vi "Temperature Bath - Simple Controller.vi"() -> ()   [LabVIEW 2023]
uses:
  <vilib>/Utility/error.llb/Trim Whitespace One-Sided.vi
  <vilib>/Instr/_visa.llb/VISA Configure Serial Port (Instr).vi
  <vilib>/Utility/file.llb/Write Delimited Spreadsheet (string).vi
panel:
  in  "stop":bool
  in  "format (%s)":string="%s"
  in  "delimiter (\\t)":string="\t"
  out "error out":errorcluster
  in  "Boolean 3":bool
  in  "VISA resource name 2":refnum<visa-resource-name>
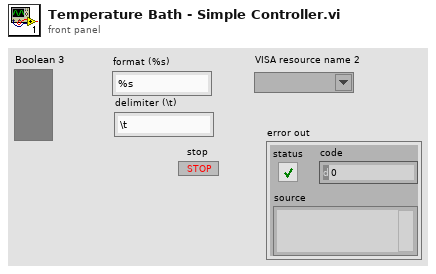
[diagram p1: front panel]
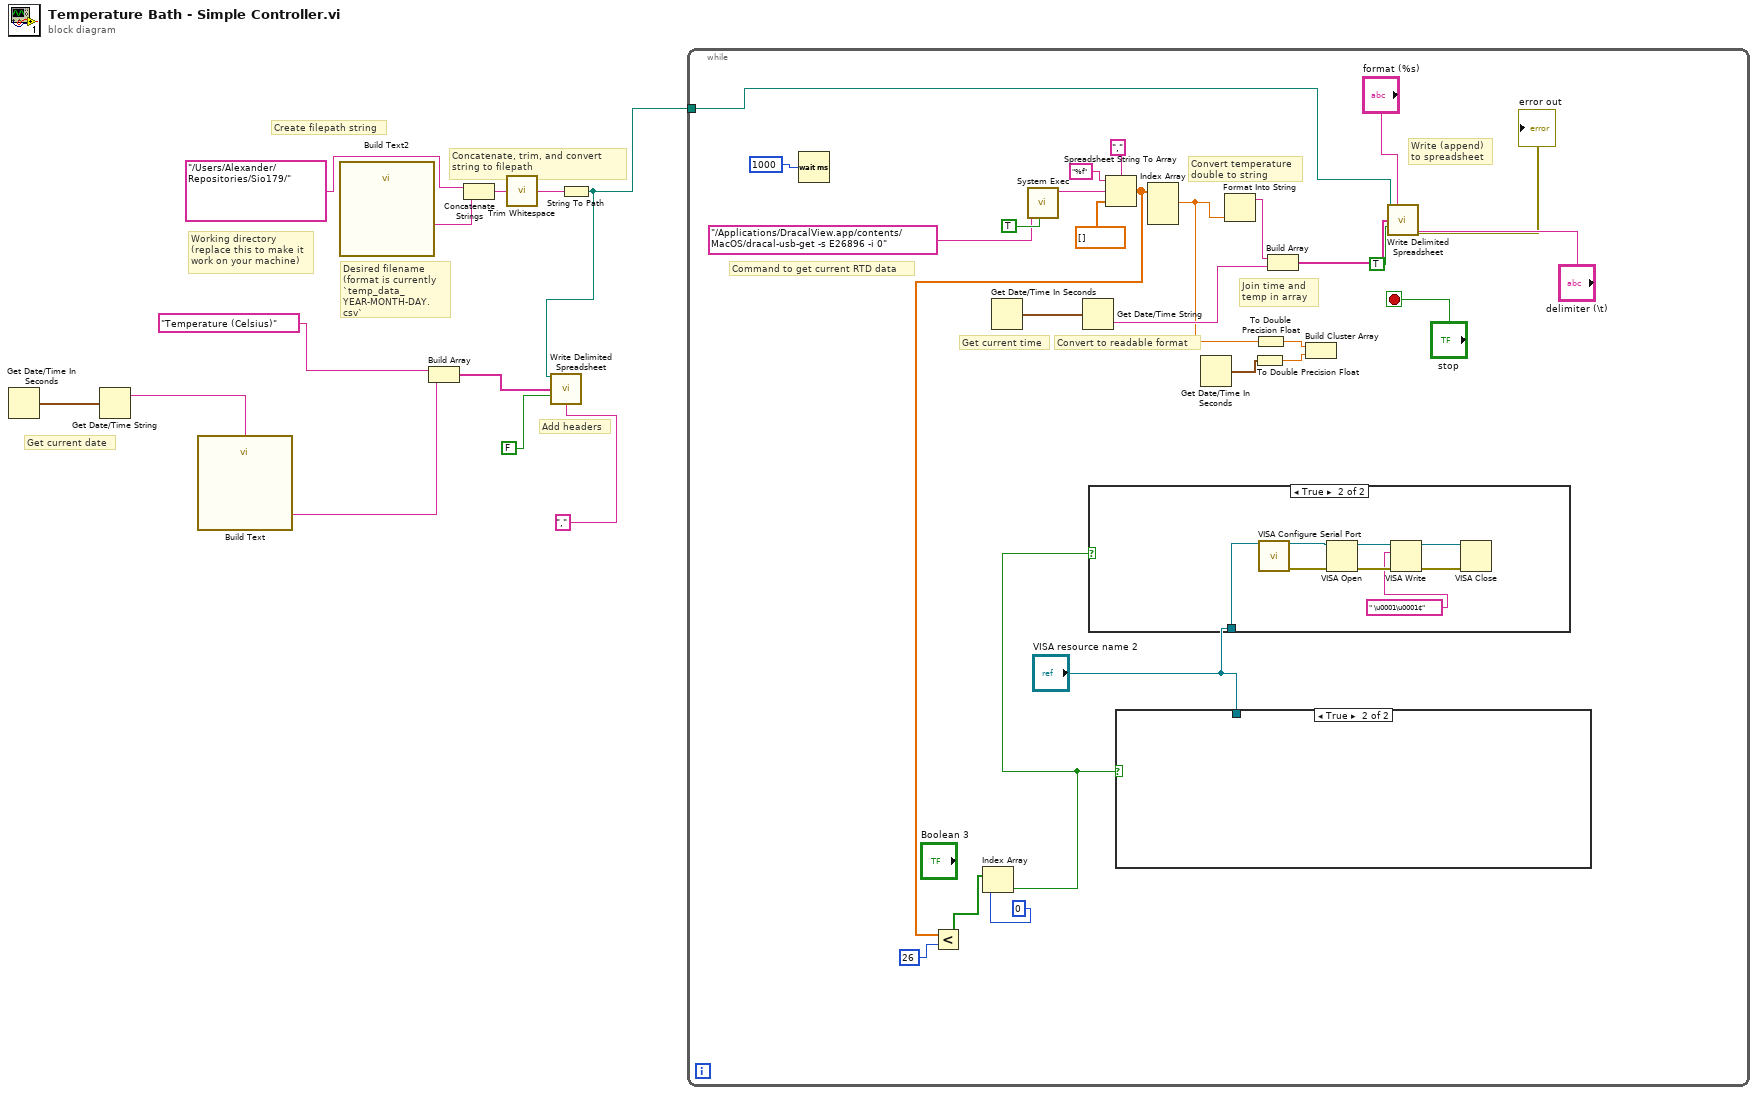
[diagram p0: block diagram]
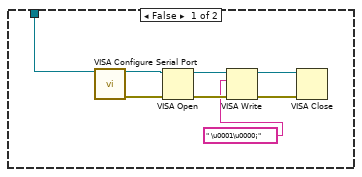
[diagram p2: hidden frame]
diagram:
  # "Add headers"
  # "Get current date"
  # "Concatenate, trim, and convert string to filepath"
  # "Desired filename (format is currently `temp_data_YEAR-MONTH-DAY.csv`"
  # "Working directory (replace this to make it work on your machine)"
  # "Create filepath string"
  n1 = Get Date/Time In Seconds() -> (seconds since 1Jan1904=w10:timestamp)
  n2 = Get Date/Time String(seconds (now)=w10) -> (date string=w6:string)  [unwired: 2 in, 1 out]
  n3 = call "Build Text"("date"=w6) -> ("Result"=w9:string)  [unwired: 13 in, 1 out]
  n4 = call "Build Text2"() -> ("Result"=w5:string)  [unwired: 14 in, 1 out]
  n5 = Build Array("Temperature (Celsius)", w9) -> (w8:string[])
  n6 = Concatenate Strings("/Users/Alexander/Repositories/Sio179/", w5) -> (w11:string)
  n7 = call <vilib>:"Trim Whitespace.vi"("string"=w11) -> ("trimmed string"=w12:string)  [unwired: 1 in]
  n8 = String To Path(string=w12) -> (path=w7:path)
  n9 = call-poly <vilib>:"Write Delimited Spreadsheet.vi"("file path (dialog if empty)"=w7, "1D data"=w8, "append to file? (new file:F)"=FALSE, "delimiter (\\t)"=",") -> ()  [unwired: 10 in, 2 out]
  n10 = while {
    tunnel: w7 -> [w23]
    stop <- "stop" stop-if-true
    # "Command to get current RTD data"
    # "Join time and temp in array"
    # "Convert temperature double to string"
    # "Convert to readable format"
    # "Get current time"
    # "Write (append) to spreadsheet"
    n11 = Wait (ms)(milliseconds to wait=u32 1000) -> ()  [unwired: 1 out]
    n12 = Get Date/Time In Seconds() -> (seconds since 1Jan1904=w32:timestamp)
    n13 = call <vilib>:"System Exec.vi"("run minimized? (F)"=TRUE, "command line"="/Applications/DracalView.app/contents/MacOS/dracal-usb-get -s E26896 -i 0") -> ("standard output"=w35:string)  [unwired: 6 in, 3 out]
    n14 = Get Date/Time String(seconds (now)=w32) -> (time string=w33:string)  [unwired: 2 in, 1 out]
    n15 = Spreadsheet String To Array(delimiter (Tab)=",", format string="%f", spreadsheet string=w35, array type (2D Dbl)=dbl[] [] ("Array")) -> (array=w18:dbl[])
    n16 = Less?(x=w18, y=26) -> (x < y?=w16:bool[])
    n17 = Index Array(array=w16, index=0) -> (element=w17:bool)
    n18 = case shown="True" w17 {
      tunnel: "VISA resource name 2" -> [_ w48]
      frame False {
      }
      frame True {
        n19 = call-poly "VISA Configure Serial Port"("VISA resource name"=w48) -> ("VISA resource name out"=w55:refnum<visa-resource-name>, "error out"=w54:errorcluster)  [unwired: 13 in]
        n20 = VISA Open(error in (no error)=w54, VISA resource name=w55) -> (VISA resource name=w53:refnum<visa-resource-name>, error out=w52:errorcluster)  [unwired: 3 in]
        n21 = VISA Write(VISA resource name=w53, write buffer=" \u0001\u0001¢", error in (no error)=w52) -> (VISA resource name out=w51:refnum<visa-resource-name>, error out=w50:errorcluster)  [unwired: 1 out]
        n22 = VISA Close(VISA resource name=w51, error in (no error)=w50) -> ()  [unwired: 1 out]
      }
    }
    n23 = case shown="True" w17 {
      tunnel: "VISA resource name 2" -> [w40 _]
      frame False {
        n24 = call-poly "VISA Configure Serial Port"("VISA resource name"=w40) -> ("VISA resource name out"=w47:refnum<visa-resource-name>, "error out"=w46:errorcluster)  [unwired: 13 in]
        n25 = VISA Open(error in (no error)=w46, VISA resource name=w47) -> (VISA resource name=w45:refnum<visa-resource-name>, error out=w44:errorcluster)  [unwired: 3 in]
        n26 = VISA Write(VISA resource name=w45, write buffer=" \u0001\u0000¡", error in (no error)=w44) -> (VISA resource name out=w43:refnum<visa-resource-name>, error out=w42:errorcluster)  [unwired: 1 out]
        n27 = VISA Close(VISA resource name=w43, error in (no error)=w42) -> ()  [unwired: 1 out]
      }
      frame True {
      }
    }
    n28 = Index Array(array=w18) -> (element #1=w22:dbl)  [unwired: 3 in, 2 out]
    n29 = Get Date/Time In Seconds() -> (seconds since 1Jan1904=w21:timestamp)
    n30 = Format Into String(w22) -> (resulting string=w24:string)  [unwired: 3 in, 1 out]
    n31 = To Double Precision Float(number=w21) -> (double precision float=w19:dbl)
    n32 = To Double Precision Float(number=w22) -> (double precision float=w20:dbl)
    n33 = Build Array(w24, w33) -> (w25:string[])
    n34 = Build Cluster Array(w20, w19) -> ()  [unwired: 1 out]
    n35 = call-poly <vilib>:"Write Delimited Spreadsheet.vi"("file path (dialog if empty)"=w23, "format (%s)"="format (%s)", "1D data"=w25, "append to file? (new file:F)"=TRUE, "delimiter (\\t)"="delimiter (\\t)") -> ("error out"=→"error out":errorcluster)  [unwired: 9 in, 1 out]
  }
